vi "Teleop.vi"(10 "Match Info":T1={"Autonomous Elapsed Seconds"=0.0, "TeleOp Elapsed Seconds"=0.0, "Disabled Elapsed Seconds"=0.0, "Visited Autonomous"=FALSE, "Visited TeleOp"=FALSE, "Visited Disabled"=FALSE, "Autonomous Settings"={"Autonomous Style"=enum."Independent", "VI Refnum"=refnum}}, 11 "Call Context":T2) -> ()   [LabVIEW 2015]
doc: "This VI is called for each TeleOp packet received from the DS where the robot is not disabled. It is often used to read from the joysticks and update I/O or to update setpoints for timed control loops. It should complete and return within 20 milliseconds or it may miss DS packets."
uses:
  <vilib>/Rock Robotics/WPI/DriverStation/WPI_DriverStationDerivedRobotMode.ctl
  <vilib>/Rock Robotics/WPI/DriverStation/WPI_DriverStationMatch Info.ctl
  <vilib>/Rock Robotics/Network Tables/NT Read Boolean.vi
  <vilib>/Rock Robotics/Network Tables/NT Read Number.vi
  <vilib>/Rock Robotics/WPI/Utilities/WPI_GetSetVariantRefNum.vi
  Robot Global Data.vi
  <vilib>/Rock Robotics/Network Tables/NT Write Boolean Array.vi
  <vilib>/Rock Robotics/Network Tables/NT Write Numeric Array.vi
panel:
  out "Sample Slider 0":dbl(slide) scale=0.0..5.0
  out "Sample Boolean 1":bool
  out "Sample Boolean 0":bool
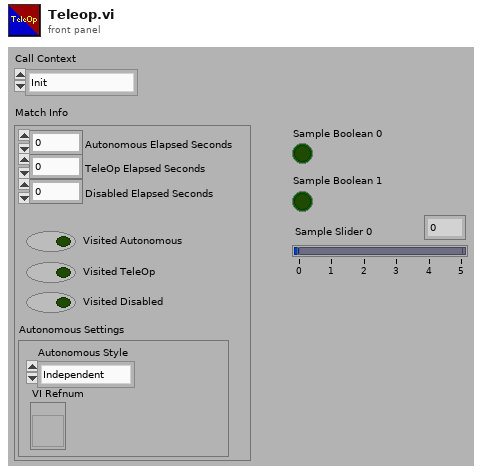
[diagram p1: front panel]
types:
  T1 = typedef "WPI_DriverStationMatch Info.ctl" = cluster{"Autonomous Elapsed Seconds":dbl, "TeleOp Elapsed Seconds":dbl, "Disabled Elapsed Seconds":dbl, "Visited Autonomous":bool, "Visited TeleOp":bool, "Visited Disabled":bool, "Autonomous Settings":cluster{"Autonomous Style":enum16{"Iterative", "Independent"}, "VI Refnum":refnum<vi>}}
  T2 = typedef "WPI_DriverStationDerivedRobotMode.ctl" = enum16{"Init", "Execute", "Stop"}
  T3 = typedef "WPI_JoystickDevRef.ctl" = cluster{"Device":T4}
  T4 = typedef "WPI_JoystickDeviceEnum.ctl" = enum16{"USB 0", "USB 1", "USB 2", "USB 3", "USB 4", "USB 5"}
  T5 = typedef "WPI_RobotDriveDevRef.ctl" = cluster{"DevStatus":errorcluster, "Motors[]":T6[], "Square Inputs":bool, "Max Output":dbl}
  T6 = typedef "WPI_MotorControlDeviceRef.ctl" = cluster{"DeviceStatus":errorcluster, "Type":T7, "PWM":cluster{"PWM Channel":T8, "DeadBand":T9}, "CAN":cluster{"Device Number":u8, "Control Mode":T10, "Semaphore":T11, "Max Vout":dbl, "TalonSRX Control Mode":T12}, "Invert":bool}
  T7 = typedef "WPI_MotorControlType.ctl" = enum16{"PWM", "CAN", "CANTalonSRX"}
  T8 = typedef "FPGA_DIOPWMChannel.ctl" = enum8{"PWM 0", "PWM 1", "PWM 2", "PWM 3", "PWM 4", "PWM 5", "PWM 6", "PWM 7", "PWM 8", "PWM 9", "PWM MXP 0", "PWM MXP 1", "PWM MXP 2", "PWM MXP 3", "PWM MXP 4", "PWM MXP 5", "PWM MXP 6", "PWM MXP 7", "PWM MXP 8", "PWM MXP 9", "Invalid"}
  T9 = typedef "WPI_PWMDeadband.ctl" = cluster{"Name":string, "maxPositivePwm":i32, "minPositivePwm":i32, "centerPwm":i32, "maxNegativePwm":i32, "minNegativePwm":i32, "angularRange":u16}
  T10 = typedef "WPI_CANJaguar_ControlMode.ctl" = enum8{"Percent VBus", "Current", "Speed", "Position", "Voltage"}
  T11 = typedef "Semaphore RefNum" = refnum<k1>
  T12 = typedef "WPI_CANTalonSRX_APIControlMode.ctl" = enum8{"Percent VBus", "Speed", "Position", "Slave", "Unchanged / Invalid", "Voltage Compensation", "Current", "Motion Profile"}
  T13 = cluster{"Buttons[0]":bool, "Buttons[1]":bool, "Buttons[2]":bool, "Buttons[3]":bool, "Buttons[4]":bool, "Buttons[5]":bool, "Buttons[6]":bool, "Buttons[7]":bool, "Buttons[8]":bool}
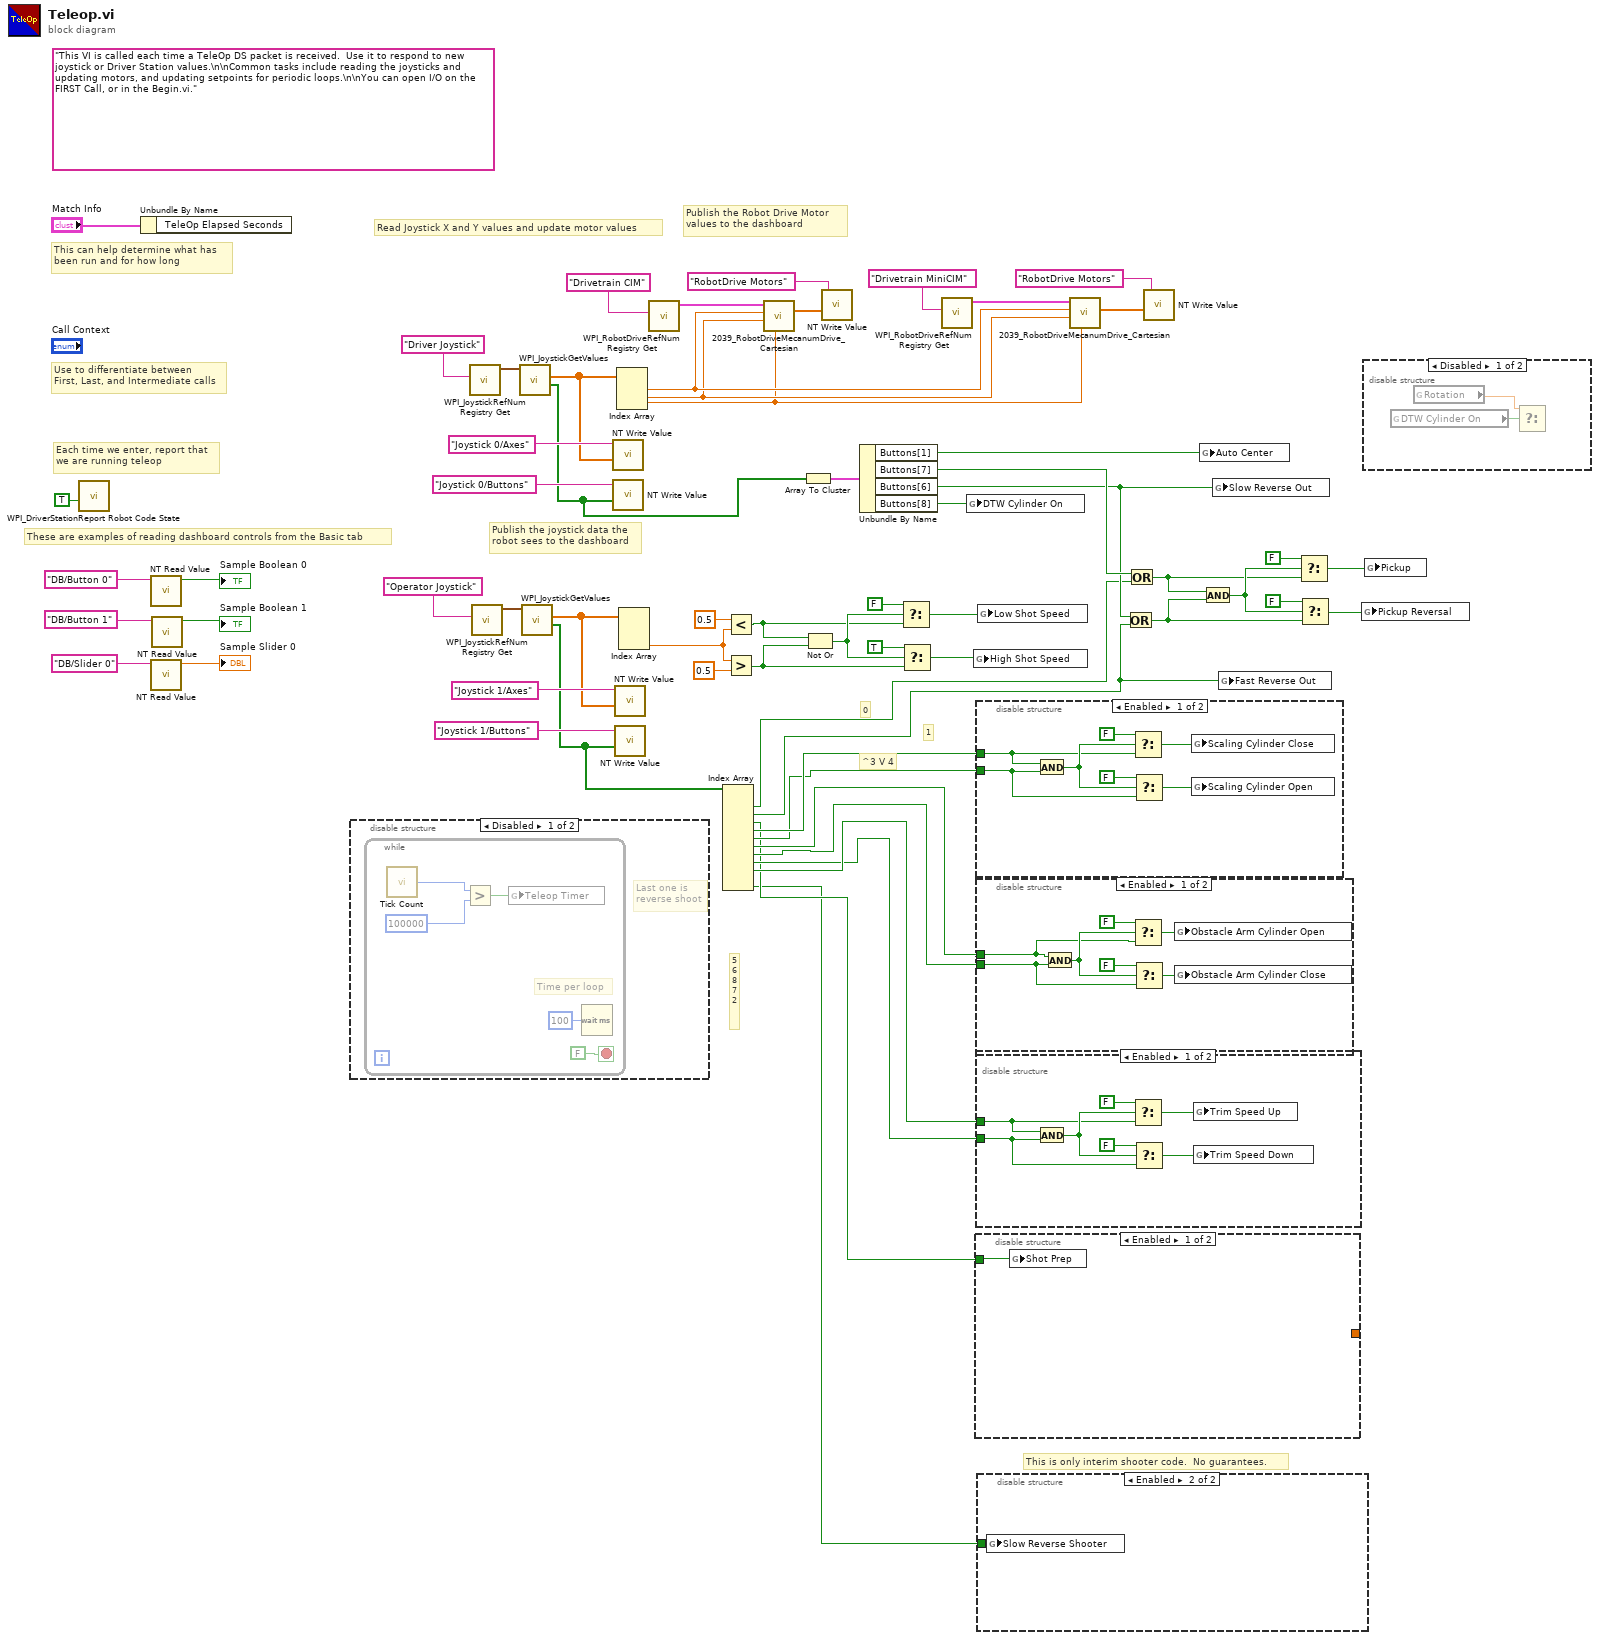
[diagram p0: block diagram]
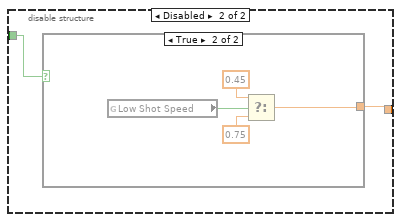
[diagram p5: hidden frame]
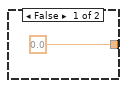
[diagram p6: hidden frame]
diagram:
  (unwired) "This VI is called each time a TeleOp DS packet is received.  Use it to respond to new joystick or Driver Station values.\n\nCommon tasks include reading the joysticks and updating motors, and updating setpoints for periodic loops.\n\nYou can open I/O on the FIRST Call, or in the Begin.vi."
  # "5\n6\n8\n7\n2"
  # "^3 V 4"
  # "1"
  # "0"
  # "This is only interim shooter code.  No guarantees."
  # "Publish the Robot Drive Motor\nvalues to the dashboard"
  # "Publish the joystick data the\nrobot sees to the dashboard"
  # "Read Joystick X and Y values and update motor values"
  # "These are examples of reading dashboard controls from the Basic tab"
  # "Each time we enter, report that\nwe are running teleop"
  # "Use to differentiate between\nFirst, Last, and Intermediate calls"
  # "This can help determine what has\nbeen run and for how long"
  n1 = call <vilib>:"WPI_DriverStationReport Robot Code State.vi"("TeleOp"=TRUE ("Autonomous")) -> ()  [unwired: 10 in, 1 out]
  n2 = Unbundle By Name("Match Info") -> ()  [unwired: 1 out]
  n3 = call-poly <vilib>:"NT Read Value.vi"("Name"="DB/Button 0" ("refnum name")) -> ("Boolean"=→"Sample Boolean 0":bool)  [unwired: 9 in, 1 out]
  n4 = call-poly <vilib>:"NT Read Value.vi"("Name"="DB/Slider 0" ("refnum name")) -> ("Numeric"=→"Sample Slider 0":dbl)  [unwired: 9 in, 1 out]
  n5 = call-poly <vilib>:"NT Read Value.vi"("Name"="DB/Button 1" ("refnum name")) -> ("Boolean"=→"Sample Boolean 1":bool)  [unwired: 9 in, 1 out]
  n6 = disable-structure shown="Disabled" {
    frame Disabled {
      # "Last one is\nreverse shoot"
      n7 = while {
        stop <- FALSE stop-if-true
        # "Time per loop"
        n8 = call "Tick Count"() -> ("Tick Count(mSec)"=w65:u32)
        n9 = Greater?(x=w65, y=u32 100000) -> (0:w64:bool)
        n10 = global write "Robot Global Data.vi" "Teleop Timer"(w64) -> ()
        n11 = Wait (ms)(milliseconds to wait=u32 100) -> ()  [unwired: 1 out]
      }
    }
    frame Enabled {
    }
  }
  n12 = call <vilib>:"WPI_JoystickRefNum Registry Get.vi"("refnum name"="Driver Joystick") -> ("JoystickDevRef"=w51:T3)  [unwired: 1 in, 9 out]
  n13 = call <vilib>:"WPI_JoystickRefNum Registry Get.vi"("refnum name"="Operator Joystick") -> ("JoystickDevRef"=w44:T3)  [unwired: 1 in, 9 out]
  n14 = call <vilib>:"WPI_JoystickGetValues.vi"("JoystickDevRef"=w51) -> ("Buttons"=w49:bool[], "Axes"=w53:dbl[])  [unwired: 6 in, 3 out]
  n15 = call <vilib>:"WPI_JoystickGetValues.vi"("JoystickDevRef"=w44) -> ("Buttons"=w14:bool[], "Axes"=w46:dbl[])  [unwired: 6 in, 3 out]
  n16 = call-poly <vilib>:"NT Write Value.vi"("Numeric Array"=w53, "Name"="Joystick 0/Axes") -> ()  [unwired: 9 in, 1 out]
  n17 = call-poly <vilib>:"NT Write Value.vi"("Boolean Array"=w49, "Name"="Joystick 0/Buttons") -> ()  [unwired: 9 in, 1 out]
  n18 = call-poly <vilib>:"NT Write Value.vi"("Numeric Array"=w46, "Name"="Joystick 1/Axes") -> ()  [unwired: 9 in, 1 out]
  n19 = call-poly <vilib>:"NT Write Value.vi"("Boolean Array"=w14, "Name"="Joystick 1/Buttons") -> ()  [unwired: 9 in, 1 out]
  n20 = Index Array(array=w53) -> (element #1=w43:dbl, element #2=w3:dbl, element #3=w2:dbl)  [unwired: 3 in]
  n21 = Index Array(array=w46) -> (element #3=w37:dbl)  [unwired: 3 in, 2 out]
  n22 = call <vilib>:"WPI_RobotDriveRefNum Registry Get.vi"("refnum name"="Drivetrain CIM") -> ("RobotDriveDevRef"=w31:T5)  [unwired: 1 in, 9 out]
  n23 = Index Array(array=w14) -> (element #1=w13:bool, element #2=w12:bool, element #3=w5:bool, element #4=w11:bool, element #5=w10:bool, element #6=w9:bool, element #7=w8:bool, element #8=w6:bool, element #9=w7:bool, element #11=w4:bool)  [unwired: 11 in, 1 out]
  n24 = Less?(x=0.5 ("y"), y=w37) -> (x < y?=w36:bool)
  n25 = Greater?(x=w37, y=0.5) -> (0:w35:bool)
  n26 = call "2039_RobotDriveMecanumDrive_Cartesian.vi"("Rotation"=w2, "Y"=w3, "X"=w43, "RobotDriveDevRef"=w31) -> ("Motor Values"=w1:dbl[])  [unwired: 5 in, 2 out]
  n27 = Array To Cluster(array=w49) -> (cluster=w50:T13)
  n28 = Not Or(1:w35, 2:w36) -> (0:w40:bool)
  n29 = call-poly <vilib>:"NT Write Value.vi"("Numeric Array"=w1, "Name"="RobotDrive Motors") -> ()  [unwired: 9 in, 1 out]
  n30 = Unbundle By Name(w50) -> ("Buttons[1]"=w15:bool, "Buttons[7]"=w18:bool, "Buttons[6]"=w16:bool, "Buttons[8]"=w17:bool)
  n31 = Select(t=FALSE, s=w40, f=w36) -> (s? t:f=w33:bool)
  n32 = Select(t=TRUE, s=w40, f=w35) -> (s? t:f=w34:bool)
  n33 = call <vilib>:"WPI_RobotDriveRefNum Registry Get.vi"("refnum name"="Drivetrain MiniCIM") -> ("RobotDriveDevRef"=w28:T5)  [unwired: 1 in, 9 out]
  n34 = global write "Robot Global Data.vi" "DTW Cylinder On"(w17) -> ()
  n35 = global write "Robot Global Data.vi" "High Shot Speed"(w34) -> ()
  n36 = disable-structure shown="Enabled" {
    disable-tunnel: w5 -> [w69 w71]
    disable-tunnel: [_ w70] -> _
    frame Enabled {
      n37 = global write "Robot Global Data.vi" "Shot Prep"(w69) -> ()
    }
    frame Disabled {
      n38 = case shown="True" w71 {
        tunnel: [0.0 w73] -> w70
        frame False {
        }
        frame True {
          n39 = global read "Robot Global Data.vi" "Low Shot Speed"() -> (w76:bool)
          n40 = Select(t=0.45, s=w76, f=0.75) -> (s? t:f=w73:dbl)
        }
      }
    }
  }
  n41 = disable-structure shown="Enabled" {
    disable-tunnel: w11 -> [w82 _]
    disable-tunnel: w10 -> [w81 _]
    frame Enabled {
      n42 = And(x=w82, y=w81) -> (x .and. y?=w83:bool)
      n43 = Select(t=FALSE, s=w83, f=w82) -> (s? t:f=w77:bool)
      n44 = Select(t=FALSE, s=w83, f=w81) -> (s? t:f=w78:bool)
      n45 = global write "Robot Global Data.vi" "Scaling Cylinder Close"(w77) -> ()
      n46 = global write "Robot Global Data.vi" "Scaling Cylinder Open"(w78) -> ()
    }
    frame Disabled {
    }
  }
  n47 = disable-structure shown="Enabled" {
    disable-tunnel: w8 -> [w85 _]
    disable-tunnel: w9 -> [w84 _]
    frame Enabled {
      n48 = And(x=w84, y=w85) -> (x .and. y?=w90:bool)
      n49 = Select(t=FALSE, s=w90, f=w84) -> (s? t:f=w86:bool)
      n50 = Select(t=FALSE, s=w90, f=w85) -> (s? t:f=w87:bool)
      n51 = global write "Robot Global Data.vi" "Obstacle Arm Cylinder Open"(w86) -> ()
      n52 = global write "Robot Global Data.vi" "Obstacle Arm Cylinder Close"(w87) -> ()
    }
    frame Disabled {
    }
  }
  n53 = disable-structure shown="Enabled" {
    disable-tunnel: w7 -> [w96 _]
    disable-tunnel: w6 -> [w95 _]
    frame Enabled {
      n54 = And(x=w96, y=w95) -> (x .and. y?=w97:bool)
      n55 = Select(t=FALSE, s=w97, f=w96) -> (s? t:f=w91:bool)
      n56 = Select(t=FALSE, s=w97, f=w95) -> (s? t:f=w92:bool)
      n57 = global write "Robot Global Data.vi" "Trim Speed Up"(w91) -> ()
      n58 = global write "Robot Global Data.vi" "Trim Speed Down"(w92) -> ()
    }
    frame Disabled {
    }
  }
  n59 = global write "Robot Global Data.vi" "Low Shot Speed"(w33) -> ()
  n60 = disable-structure shown="Enabled" {
    disable-tunnel: w4 -> [_ w98]
    frame Disabled {
    }
    frame Enabled {
      n61 = global write "Robot Global Data.vi" "Slow Reverse Shooter"(w98) -> ()
    }
  }
  n62 = call "2039_RobotDriveMecanumDrive_Cartesian.vi"("Rotation"=w2, "Y"=w3, "X"=w43, "RobotDriveDevRef"=w28) -> ("Motor Values"=w27:dbl[])  [unwired: 5 in, 2 out]
  n63 = Or(x=w16, y=w12) -> (x .or. y?=w19:bool)
  n64 = Or(x=w18, y=w13) -> (x .or. y?=w20:bool)
  n65 = call-poly <vilib>:"NT Write Value.vi"("Numeric Array"=w27, "Name"="RobotDrive Motors") -> ()  [unwired: 9 in, 1 out]
  n66 = global write "Robot Global Data.vi" "Auto Center"(w15) -> ()
  n67 = And(x=w20, y=w19) -> (x .and. y?=w25:bool)
  n68 = global write "Robot Global Data.vi" "Slow Reverse Out"(w16) -> ()
  n69 = global write "Robot Global Data.vi" "Fast Reverse Out"(w12) -> ()
  n70 = Select(t=FALSE, s=w25, f=w20) -> (s? t:f=w22:bool)
  n71 = Select(t=FALSE, s=w25, f=w19) -> (s? t:f=w21:bool)
  n72 = global write "Robot Global Data.vi" "Pickup Reversal"(w21) -> ()
  n73 = disable-structure shown="Disabled" {
    frame Disabled {
      n74 = global read "Robot Global Data.vi" "DTW Cylinder On"() -> (w101:bool)
      n75 = global read "Robot Global Data.vi" "Rotation"() -> (w100:dbl)
      n76 = Select(t=w100, s=w101) -> (f=w99:dbl)  [unwired: 1 out]
    }
    frame Enabled {
    }
  }
  n77 = global write "Robot Global Data.vi" "Pickup"(w22) -> ()
